vi "Close.vi"(4 "error in (no error)":errorcluster, 7 "Device handle":u32 format="%x") -> (0 "error out":errorcluster)   [LabVIEW 2014, in "MBUG-2820.lvlib"]
doc: "Close the connection to the device. Thedevice can not be accessed afterwards."
uses:
  <instrlib>/MBUG-2820/MBUG-2820.lvlib
  <instrlib>/MBUG-2820/mbugdll.dll
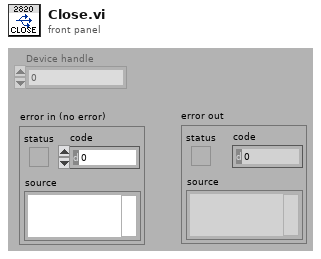
[diagram p1: front panel]
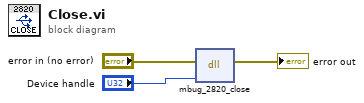
[diagram p0: block diagram]
diagram:
  n1 = dll-call lib="C:/Programme/National Instruments/LabVIEW 2014/instr.lib/MBUG-2820/mbugdll.dll" fn="mbug_2820_close"(error in="error in (no error)", "dev_handle"="Device handle") -> (error out=→"error out":errorcluster)  [unwired: 4 in, 1 out]
